vi "CurrRefFres.vi"() -> ()   [LabVIEW 2014]
uses:
  <vilib>/rvi/eio/common/nirviEmuTemplateMethod_errors.vi
  <vilib>/eio/EIONode/EIONode.xnode
panel:
  out "Finished?":bool
  out "Ref":sgl
  in  "SampleNum":i32
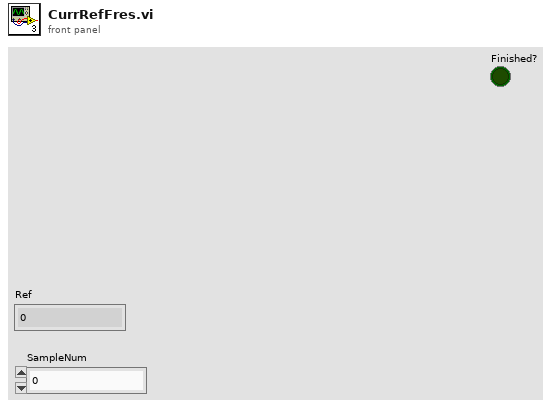
[diagram p1: front panel]
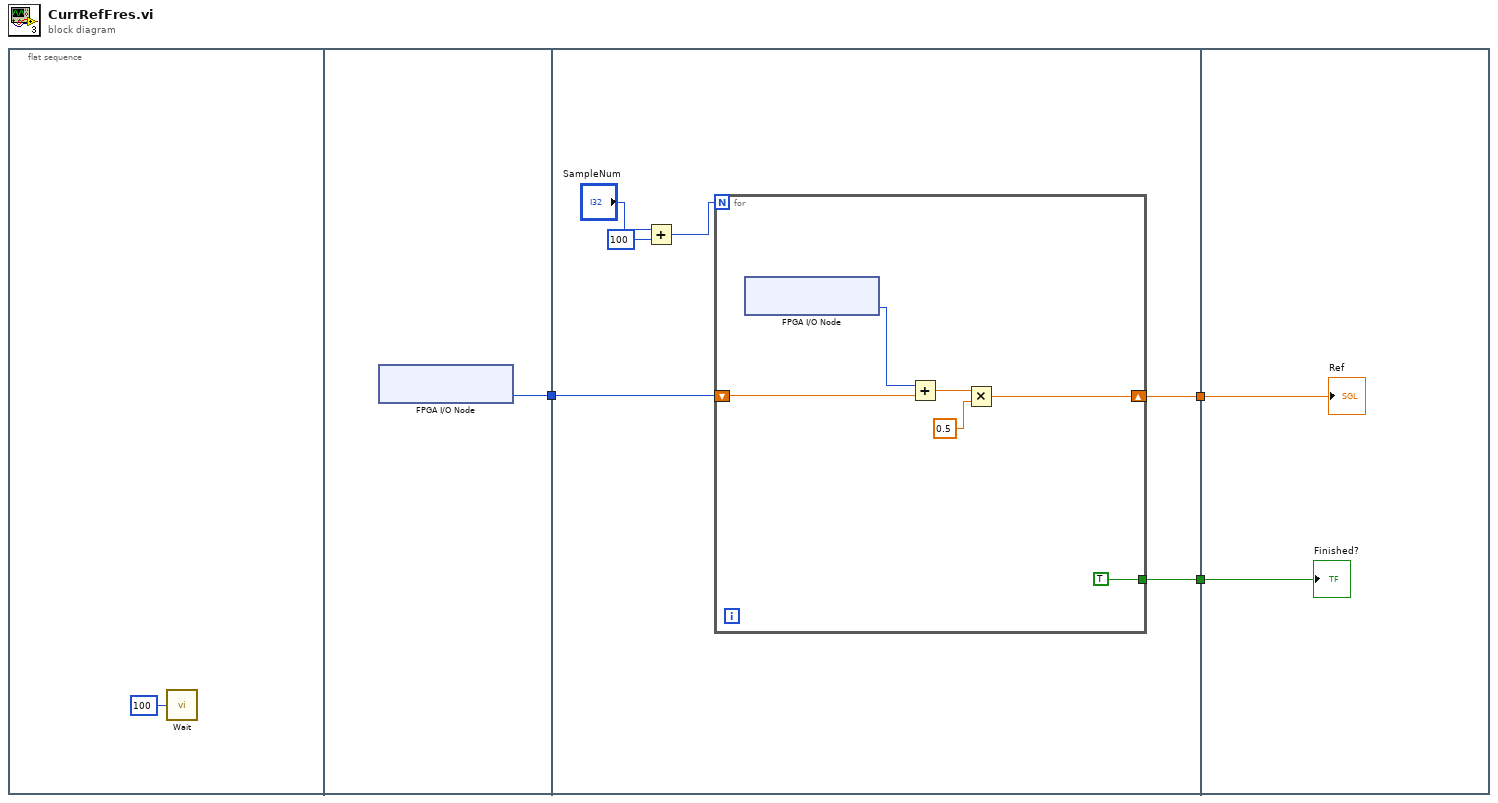
[diagram p0: block diagram]
diagram:
  n1 = flat-sequence {
    tunnel: [w5] -> w3
    tunnel: w3 -> [w11]
    tunnel: [w10] -> w2
    tunnel: [w9] -> w1
    tunnel: w2 -> [w19]
    tunnel: w1 -> [w18]
    frame #0 {
      n2 = call "Wait"("Count(uSec)"=u32 100) -> ()  [unwired: 1 out]
    }
    frame #1 {
      n3 = xnode "FPGA I/O Node"() -> ("Connector0/AI1"=w5:i16)  [unwired: 1 in, 1 out]
    }
    frame #2 {
      n4 = Add(x="SampleNum", y=100) -> (x+y=w6:i32)
      n5 = for {
        N: w6 -> [_]
        shift-right: [w13] -> w10
        shift-left: w11 -> [w16]
        tunnel: [TRUE] -> w9
        n6 = xnode "FPGA I/O Node"() -> ("Connector0/AI1"=w17:i16)  [unwired: 1 in, 1 out]
        n7 = Add(x=w17, y=w16) -> (x+y=w15:sgl)
        n8 = Multiply(x=w15, y=sgl 0.5) -> (x*y=w13:sgl)
      }
    }
    frame #3 {
      "Ref" <- w19
      "Finished?" <- w18
    }
  }
